vi "Set Initialization Data - SDAQ.vi"(8 "error in":errorcluster, 11 "UserInterface in":refnum<class "UserInterface.lvclass">) -> (0 "error out":errorcluster, 3 "UserInterface out":refnum<class "UserInterface.lvclass">)   [LabVIEW 2021, in "UserInterface.lvclass"]
doc: "Sets the initialization data of a statically linked subWorker."
uses:
  UserInterface.lvclass
  C:/Program Files (x86)/National Instruments/LabVIEW 2021/vi.lib/addons/_Workers/Library/Classes/Worker/Worker.lvclass
  SimulationDaq/Initialization Data.ctl
  <vilib>/addons/_Workers/Library/Classes/Message Queue/Message Queue.lvclass
  <vilib>/addons/_Workers/Library/Case Label.ctl
  UserInterface.lvclass/UserInterface.ctl
  <vilib>/addons/_Workers/Library/Classes/Worker/Worker.lvclass/Worker.ctl
  SimulationDaq/SimulationDaq.lvclass
  <vilib>/addons/_Workers/Library/Workers.lvlib
  <vilib>/addons/_Workers/Library/Classes/Worker/Worker.lvclass
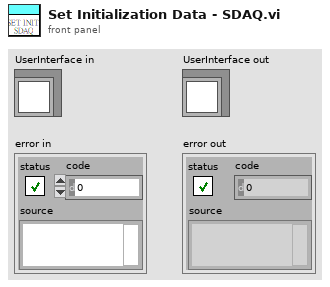
[diagram p1: front panel]
types:
  T1 = typedef "SimulationDaq.lvclass/Initialization Data.ctl" = cluster{"CallerEnQ":refnum<class "Message Queue.lvclass">, "ReturnCaseLabel":T2}
  T2 = typedef "Workers.lvlib/Case Label.ctl" = string
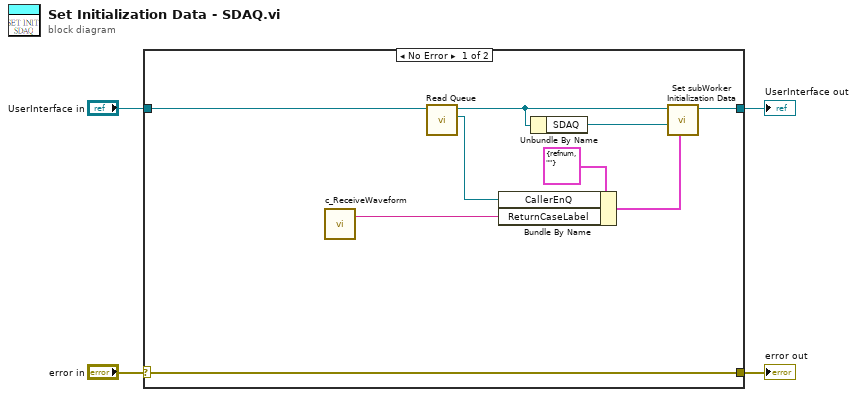
[diagram p0: block diagram]
diagram:
  n1 = case shown="No Error" "error in" {
    selector: "error in" -> [w13 w15]
    tunnel: [w13 w15] -> w3
    tunnel: [w11 w14] -> w2
    tunnel: "UserInterface in" -> [w10 w14]
    frame No Error {
      n2 = call "c_ReceiveWaveform.vi"() -> ("Case Label"=w7:T2)  [unwired: 1 in]
      n3 = call <vilib>:"Read Queue.vi"("Worker"=w10) -> ("Message Queue out"=w8:refnum<class "Message Queue.lvclass">, "dup Worker out"=w9:refnum<class "UserInterface.lvclass">)  [unwired: 9 in]
      n4 = Bundle By Name(cluster=T1 {"CallerEnQ"=refnum, "ReturnCaseLabel"=""} ("Initialization Data"), "CallerEnQ"=w8, "ReturnCaseLabel"=w7) -> (w5:T1)
      n5 = Unbundle By Name(w9) -> ("SDAQ"=w12:refnum<class "SimulationDaq.lvclass">)
      n6 = call-dynamic "Set subWorker Initialization Data.vi"("Initialization Data"=w5, "subWorker"=w12, "Worker"=w9) -> ("Worker out"=w11:refnum<class "UserInterface.lvclass">)  [unwired: 8 in]
    }
    frame Error {
    }
  }
  "error out" <- w3
  "UserInterface out" <- w2
